vi "XML_FF_readTrial.vi"(8 "error in (no error)":errorcluster, 10 "Trial Number":i32, 11 "DOM document in":refnum<k20>) -> (0 "error out":errorcluster, 2 "Trial out":T1, 3 "DOM document out":refnum<k20>)   [LabVIEW 2016, in "XML_EEG_Features.lvlib"]
doc: "Прочитать пробу из XML файла, содержащего рассчитанные значения спектра сигнала ЭЭГ"
uses:
  XML_EEG_Features.lvlib
  XML_FF_Trial.ctl
  <vilib>/xml/NI_XML.lvlib
panel:
  # "This VI is a part of BCI Design library, http://www.ru-bci.org \nCopyright © 2020, Sotnikov Peter, All rights reserved. License: CC BY-NC 4.0"
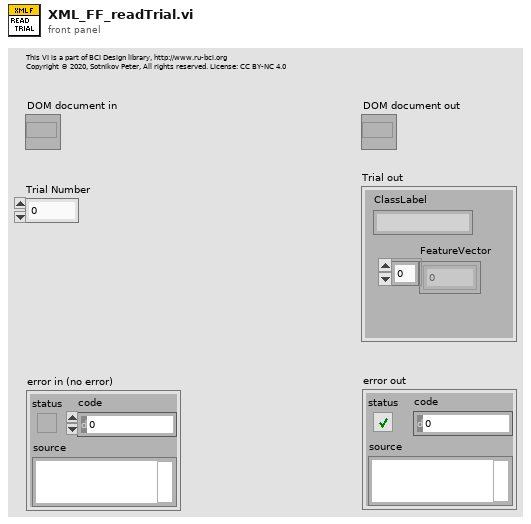
[diagram p1: front panel]
types:
  T1 = typedef "XML_EEG_Features.lvlib/XML_FF_Trial.ctl" = cluster{"ClassLabel":string, "FeatureVector":dbl[]}
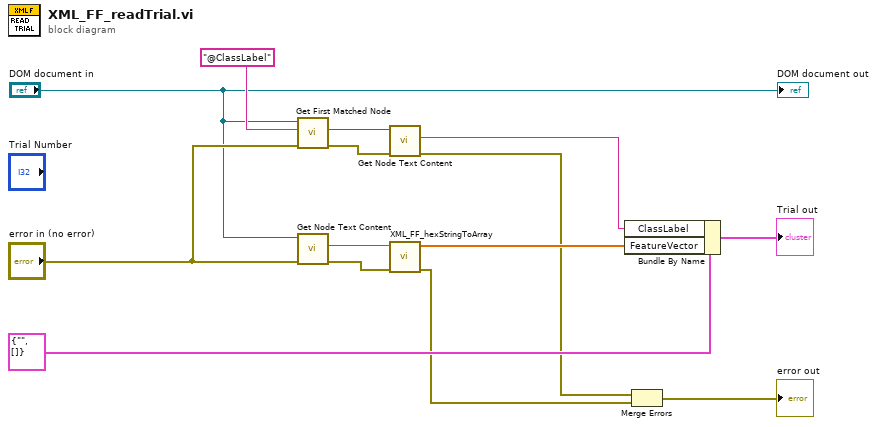
[diagram p0: block diagram]
diagram:
  n1 = call <vilib>:"Get First Matched Node.vi"("error in (no error)"="error in (no error)", "XPath expression"="@ClassLabel", "node in"="DOM document in") -> ("error out"=w8:errorcluster, "node result"=w7:refnum<k20>)  [unwired: 6 in, 1 out]
  n2 = call <vilib>:"Get Node Text Content.vi"("error in (no error)"="error in (no error)", "node in"="DOM document in") -> ("error out"=w1:errorcluster, "node text"=w4:string)  [unwired: 7 in, 1 out]
  n3 = call <vilib>:"Get Node Text Content.vi"("error in (no error)"=w8, "node in"=w7) -> ("error out"=w6:errorcluster, "node text"=w5:string)  [unwired: 7 in, 1 out]
  n4 = call "XML_FF_hexStringToArray.vi"("error in (no error)"=w1, "Hex String in"=w4) -> ("error out"=w11:errorcluster, "Array out"=w12:dbl[])  [unwired: 8 in]
  n5 = Bundle By Name(cluster=T1 {"ClassLabel"="", "FeatureVector"=[]} ("XML_FF_Trial"), "ClassLabel"=w5, "FeatureVector"=w12) -> (→"Trial out":T1)
  n6 = Merge Errors(w6, w11) -> (→"error out":errorcluster)
  "DOM document out" <- "DOM document in"
